vi "checkDataType.vi"(9 "Data":variant, 10 "DataType":variant) -> (0 "error out":errorcluster, 2 "Data out":variant)   [LabVIEW 2025, in "ObserverClass.lvlib"]
doc: "Check if input Data Type are equal"
uses:
  ObserverClass.lvlib
  <vilib>/Utility/Data Type/NI_Data Type.lvlib
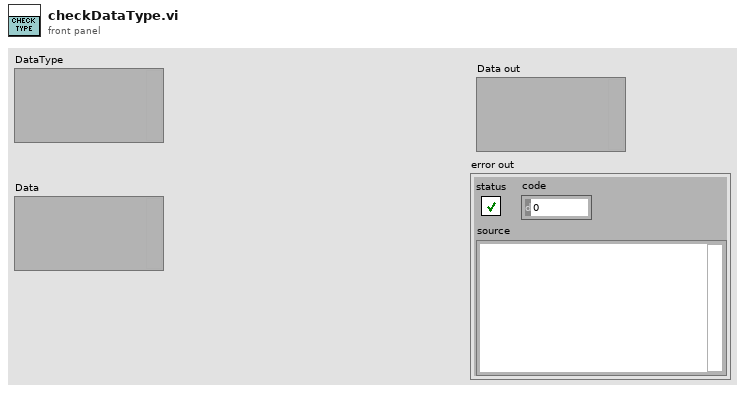
[diagram p1: front panel]
types:
  T1 = typedef "NI_Data Type.lvlib/Data Type.ctl" = enum8{"Invalid Type", "Void", "I8", "I16", "I32", "I64", "U8", "U16", "U32", "U64", "Single Float", "Double Float", "Extended Float", "Single Complex", "Double Complex", "Extended Complex", "Enum U8", "Enum U16", "Enum U32", "Enum U64", "Single Float With Unit", "Double Float With Unit", "Extended Float With Unit", "Single Complex with Unit", "Double Complex with Unit", "Extended Complex with Unit", "Boolean", "String", "Path", "Picture", "Tag", "Array", "Cluster", "Variant", "LV Variant", "Waveform", "Timestamp", "Digital Waveform", "Digital Data", "ExpressData", "Refnum", "External Data", "VI", "Poly VI", "LabVIEW Class Instance", "Fixed Point", "Set Collection", "Map Collection"}
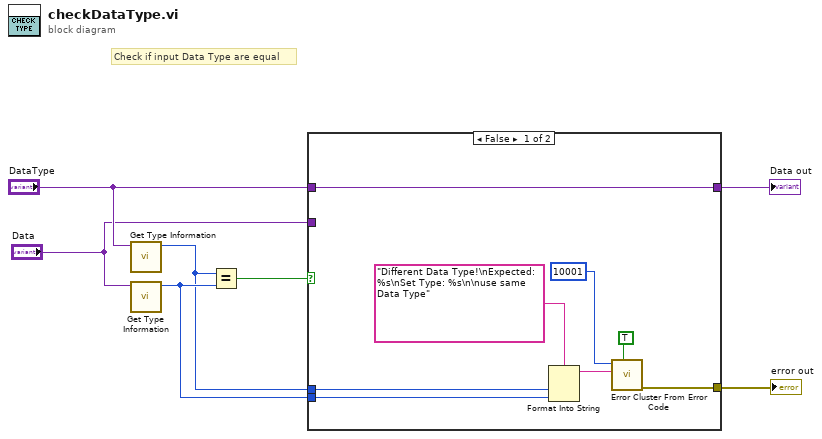
[diagram p0: block diagram]
diagram:
  # "Check if input Data Type are equal"
  n1 = call <vilib>:"Get Type Information.vi"("variant"="DataType") -> ("type"=w1:T1)  [unwired: 6 in, 4 out]
  n2 = call <vilib>:"Get Type Information.vi"("variant"="Data") -> ("type"=w2:T1)  [unwired: 6 in, 4 out]
  n3 = Equal?(x=w1, y=w2) -> (x = y?=w3:bool)
  n4 = case shown="False" w3 {
    tunnel: [w15 _] -> w7
    tunnel: "DataType" -> [w11 _]
    tunnel: "Data" -> [_ w16]
    tunnel: [w11 w16] -> w6
    tunnel: w2 -> [w9 _]
    tunnel: w1 -> [w8 _]
    frame False {
      n5 = Format Into String(format string="Different Data Type!\nExpected: %s\nSet Type: %s\n\nuse same Data Type", w8, w9) -> (resulting string=w13:string)  [unwired: 2 in, 1 out]
      n6 = call <vilib>:"Error Cluster From Error Code.vi"("show call chain? (False)"=TRUE, "error message (\"\")"=w13, "error code (0)"=10001) -> ("error out"=w15:errorcluster)  [unwired: 6 in]
    }
    frame True {
    }
  }
  "error out" <- w7
  "Data out" <- w6
